vi "Write_error_to_error_indicator.vi"(1 "From unit number(0)":u8, 2 "error message":string, 3 "Error string indicator reference":refnum<vi>) -> ()   [LabVIEW 2013]
panel:
  out "String out":string
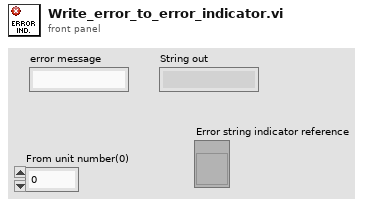
[diagram p1: front panel]
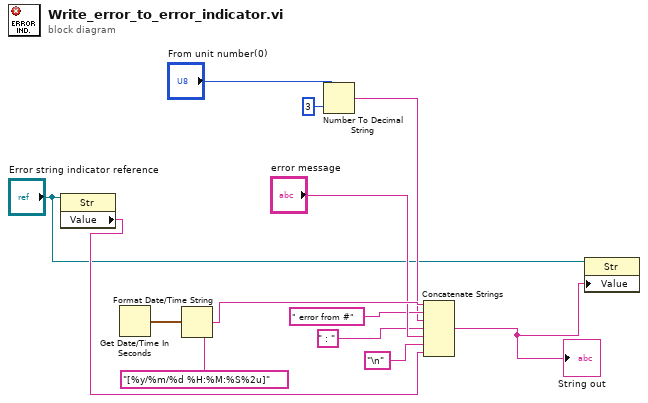
[diagram p0: block diagram]
diagram:
  n1 = property on="Property Node" class="Str"(reference="Error string indicator reference") -> ("Value"=w6:string)  [unwired: 1 in, 2 out]
  n2 = Get Date/Time In Seconds() -> (seconds since 1Jan1904=w11:timestamp)
  n3 = Format Date/Time String(time format string (%c)="[%y/%m/%d %H:%M:%S%2u]", seconds (now)=w11) -> (date/time string=w12:string)  [unwired: 1 in]
  n4 = Number To Decimal String(number="From unit number(0)", width (-)=i16 3) -> (decimal integer string=w3:string)
  n5 = Concatenate Strings(w12, " error from #" ("string"), w3, " : " ("string"), "error message", "\n" ("string"), w6) -> (w5:string)
  "String out" <- w5
  n6 = property on="Property Node" class="Str"(reference="Error string indicator reference", "Value"=w5) -> ()  [unwired: 1 in, 2 out]
